vi "Get Path Regex.vi"(8 "error in (no error)":errorcluster, 11 "QueryAuthController in":refnum<class "QueryAuthController.lvclass">) -> (0 "error out":errorcluster, 2 "Path Regex":string, 3 "QueryAuthController out":refnum<class "QueryAuthController.lvclass">)   [LabVIEW 2020, in "QueryAuthController.lvclass"]
uses:
  QueryAuthController.lvclass
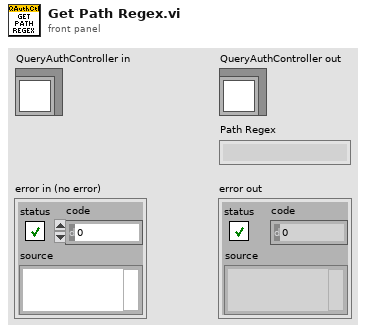
[diagram p1: front panel]
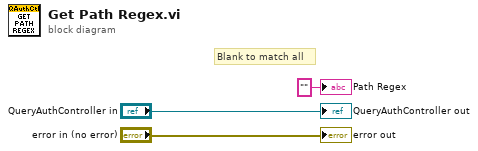
[diagram p0: block diagram]
diagram:
  # "Blank to match all"
  "error out" <- "error in (no error)"
  "QueryAuthController out" <- "QueryAuthController in"
  "Path Regex" <- "" ("Path Regex")
